vi "Stop PIS Loops_Asylum.vi"(10 "PIS Loop Number (0-5)":u32 max=5 step=1) -> (2 "error out":errorcluster)   [LabVIEW 2016]
doc: "This VI turn off the specified PIDS loop (0~5)."
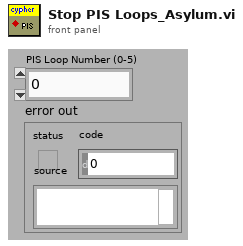
[diagram p1: front panel]
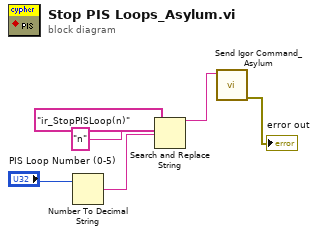
[diagram p0: block diagram]
diagram:
  n1 = Number To Decimal String(number="PIS Loop Number (0-5)") -> (decimal integer string=w3:string)  [unwired: 1 out]
  n2 = Search and Replace String(input string="ir_StopPISLoop(n)", search string="n", replace string=w3) -> (result string=w2:string)  [unwired: 1 in, 7 out]
  n3 = call "Send Igor Command_Asylum.vi"("Command"=w2) -> ("error out"=→"error out":errorcluster)  [unwired: 7 in, 2 out]
